vi "XY Set Control Enable State.vi"(8 "error in (no error)":errorcluster, 10 "Enabled?":bool=TRUE, 11 "Controls":refnum<vi>[](array[refnum])) -> (0 "error out":errorcluster)   [LabVIEW 2012, in "Workspace MultiY Graph.lvlib"]
uses:
  Workspace MultiY Graph.lvlib
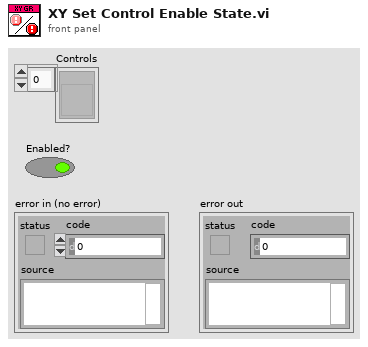
[diagram p1: front panel]
types:
  T1 = enum8{"Enabled", "Disabled", "Disabled and Grayed Out"}
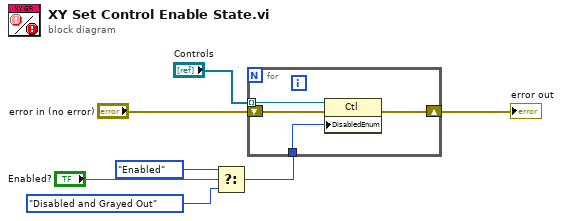
[diagram p0: block diagram]
diagram:
  n1 = Select(t=T1."Enabled" ("Disabled"), s="Enabled?", f=T1."Disabled and Grayed Out" ("Disabled")) -> (s? t:f=w2:T1)
  n2 = for {
    tunnel: "Controls" -> [w10] mode=indexing
    shift-right: [w9] -> w7
    shift-left: "error in (no error)" -> [w11]
    tunnel: w2 -> [w8]
    n3 = property class="Ctl"(reference=w10, error in=w11, "DisabledEnum"=w8) -> (error out=w9:errorcluster)  [unwired: 1 out]
  }
  "error out" <- w7
